vi "DHTxx_Initial.vi"(8 "error in (no error)":errorcluster) -> (0 "error out":errorcluster, 3 "return type":i32)   [LabVIEW 2014, in "QwaveSys RPi Training Library.lvlib"]
uses:
  <vilib>/Q-Wave Systems/QwaveSys RPi Package 2.0/Addons/QwaveSys RPi Training Library.lvlib
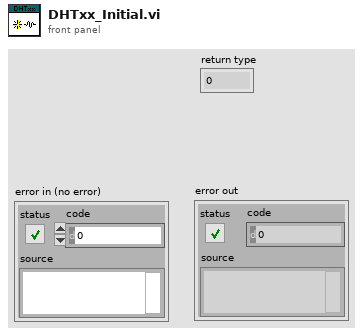
[diagram p1: front panel]
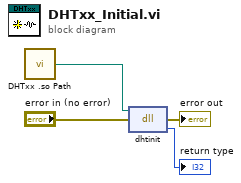
[diagram p0: block diagram]
diagram:
  n1 = call <vilib>:"DHTxx .so Path.vi"() -> ("DHTxx .so Path"=w1:path)  [unwired: 5 in]
  n2 = dll-call lib="libdht.so" fn="dhtinit"(path in=w1, error in="error in (no error)") -> (error out=→"error out":errorcluster, "return type"=→"return type":i32)  [unwired: 1 in, 1 out]
